vi "MessageGui.vi"(8 "error in":errorcluster, 10 "Message":string) -> (0 "error out":errorcluster)   [LabVIEW 2019, in "Tools.lvlib"]
uses:
  Tools.lvlib
  controls/buttons/OK.ctl
  MessageGui.Action.ctl
panel:
  out "_loop":i32(ring)=4
  in  "OKButton":T1
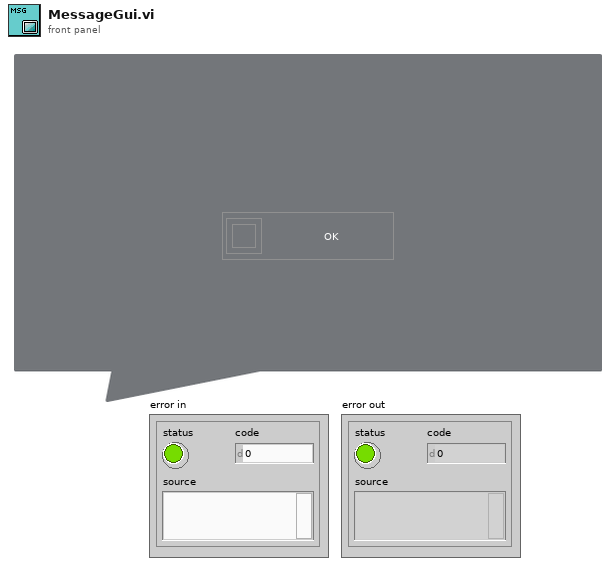
[diagram p1: front panel]
types:
  T1 = typedef "Tools.lvlib/OK.ctl" = bool
  T2 = typedef "Tools.lvlib/MessageGui.Action.ctl" = enum32{"idle", "constructor", "destructor", "--- MessageGUI ---", "Gui.Translate"}
  T3 = enum32{"invalid app kind", "Development System", "Run Time System", "Student Edition", "Embedded LabVIEW", "Evaluation", "Custom"}
  T4 = typedef "LVPositionTypeDef.ctl" = cluster{"Left":i32, "Top":i32}
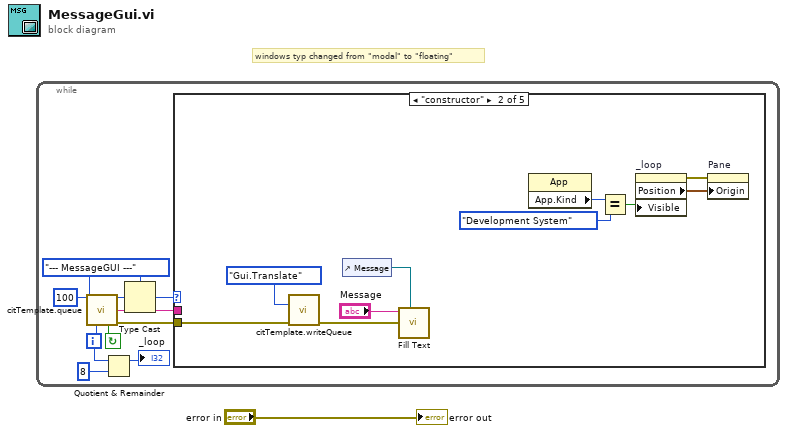
[diagram p0: block diagram]
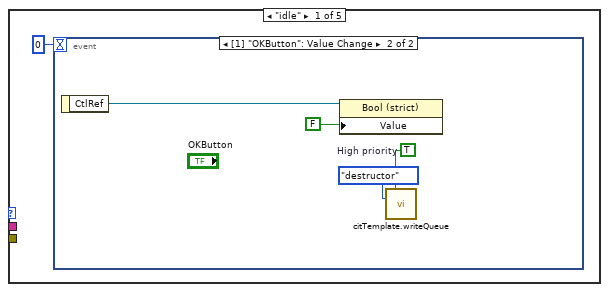
[diagram p2: hidden frame]
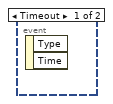
[diagram p3: hidden frame]
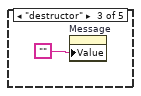
[diagram p4: hidden frame]
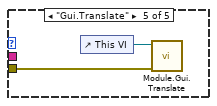
[diagram p6: hidden frame]
diagram:
  # "windows typ changed from \"modal\" to \"floating\""
  n1 = while {
    i -> [w2]
    stop <- w11 continue-if-true
    w5 = MessageGui.Action."--- MessageGUI ---" ("Action")
    n2 = call "citTemplate.queue.vi"("ms timeout (250 ms)"=100, "event enum"=w5, "iteration (-1)"=w2) -> ("event out"=w9:u32, "(flatten) data out"=w6:string, "continue"=w11:bool, "error out"=w7:errorcluster)  [unwired: 2 in, 7 out]
    n3 = Quotient & Remainder(x=w2, y=8) -> (x-y*floor(x/y)=→"_loop":i32)  [unwired: 1 out]
    n4 = Type Cast(type=w5, x=w9) -> (*(type *) &x=w8:T2)
    n5 = case shown="\"constructor\"" w8 {
      tunnel: w7 -> [_ w21 _ _ w28]
      tunnel: w6 -> [_ _ _ _ _]
      frame "idle" {
        n6 = event shown="[1] \"OKButton\": Value Change" {
          selector: _ -> [_ _]
          dyn-events: _ -> [_ _]
          timeout: 0 -> [_ _]
          event Timeout {
            n7 = event-data() -> ()  [unwired: 3 out]
          }
          event Value Change {
            w13 = TRUE  # High priority
            n8 = event-data() -> ("CtlRef"=w15:refnum<vi>)  [unwired: 1 out]
            n9 = property class="Bool (strict)"(reference=w15, "Value"=T1 FALSE) -> ()  [unwired: 1 in, 2 out]
            n10 = call "citTemplate.writeQueue.vi"("High priority (F)"=w13, "event in (if not connected:all statemachine with data event)"=MessageGui.Action."destructor" ("Action")) -> ()  [unwired: 3 in, 11 out]
          }
        }
      }
      frame "constructor" {
        n11 = call "citTemplate.writeQueue.vi"("event in (if not connected:all statemachine with data event)"=MessageGui.Action."Gui.Translate" ("Action"), "error in (no error)"=w21) -> ("error out"=w18:errorcluster)  [unwired: 13 in]
        n12 = control-ref of="Message"() -> (w19:refnum<vi>)
        n13 = call "Fill Text.vi"("String ref"=w19, "Error In"=w18, "String in"="Message") -> ()  [unwired: 8 in, 1 out]
        n14 = property class="App"() -> ("App.Kind"=w24:T3)  [unwired: 2 in, 2 out]
        n15 = Equal?(x=w24, y=T3."Development System") -> (x = y?=w22:bool)
        n16 = property on="_loop" class="Ring (strict)"("Visible"=w22) -> (error out=w25:errorcluster, "Position"=w26:T4)  [unwired: 2 in, 1 out]
        n17 = property on="Pane" class="Pane"(error in=w25, "Origin"=w26) -> ()  [unwired: 1 in, 2 out]
      }
      frame "destructor" {
        n18 = property on="Message" class="Str"("Value"="") -> ()  [unwired: 2 in, 2 out]
      }
      frame "--- MessageGUI ---" {
      }
      frame "Gui.Translate" {
        n19 = control-ref of="This VI"() -> (w29:refnum<vi>)
        n20 = call "Module.Gui.Translate.vi"("error in"=w28, "VI ref in"=w29) -> ()  [unwired: 7 in, 3 out]
      }
    }
  }
  "error out" <- "error in"
